vi "F510-X.vi"(8 "error in (no error)":errorcluster, 10 "Deadzone Scale Cluster":cluster{"Scale":dbl, "Deadzone":dbl}={"Scale"=1.0, "Deadzone"=0.1}, 11 "refnum name":string) -> (0 "error out":errorcluster, 1 "Right Stick":cluster{"X":dbl, "Y":dbl}, 2 "Left Stick":cluster{"X":dbl, "Y":dbl}, 3 "JoystickDevRef":T2, 4 "Buttons":T1, 5 "Triggers":cluster{"Left":dbl, "Right":dbl}, 6 "D-Pad Buttons":T4)   [LabVIEW 2014]
uses:
  <vilib>/Rock Robotics/WPI/Joystick/WPI_JoystickDevRef.ctl
  <vilib>/Rock Robotics/WPI/Joystick/WPI_JoystickDeviceEnum.ctl
  <vilib>/Rock Robotics/WPI/Joystick/WPI_JoystickGetSetRefNum.vi
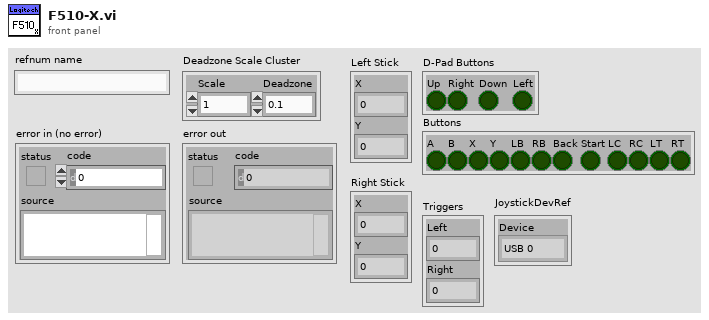
[diagram p1: front panel]
types:
  T1 = cluster{"A":bool, "B":bool, "X":bool, "Y":bool, "LB":bool, "RB":bool, "Back":bool, "Start":bool, "LC":bool, "RC":bool, "LT":bool, "RT":bool}
  T2 = typedef "WPI_JoystickDevRef.ctl" = cluster{"Device":T3}
  T3 = typedef "WPI_JoystickDeviceEnum.ctl" = enum16{"USB 0", "USB 1", "USB 2", "USB 3", "USB 4", "USB 5"}
  T4 = cluster{"Up":bool, "Right":bool, "Down":bool, "Left":bool}
  T5 = cluster{"[0]":dbl, "[1]":dbl, "[2]":dbl, "[3]":dbl, "[4]":dbl, "[5]":dbl}
  T6 = cluster{"Buttons[0]":bool, "Buttons[1]":bool, "Buttons[2]":bool, "Buttons[3]":bool, "Buttons[4]":bool, "Buttons[5]":bool, "Buttons[6]":bool, "Buttons[7]":bool, "Buttons[8]":bool, "Buttons[9]":bool}
  T7 = cluster{"Up":bool, "Down":bool, "Left":bool, "Right":bool}[]
  T8 = cluster{"Up":bool, "Down":bool, "Left":bool, "Right":bool}
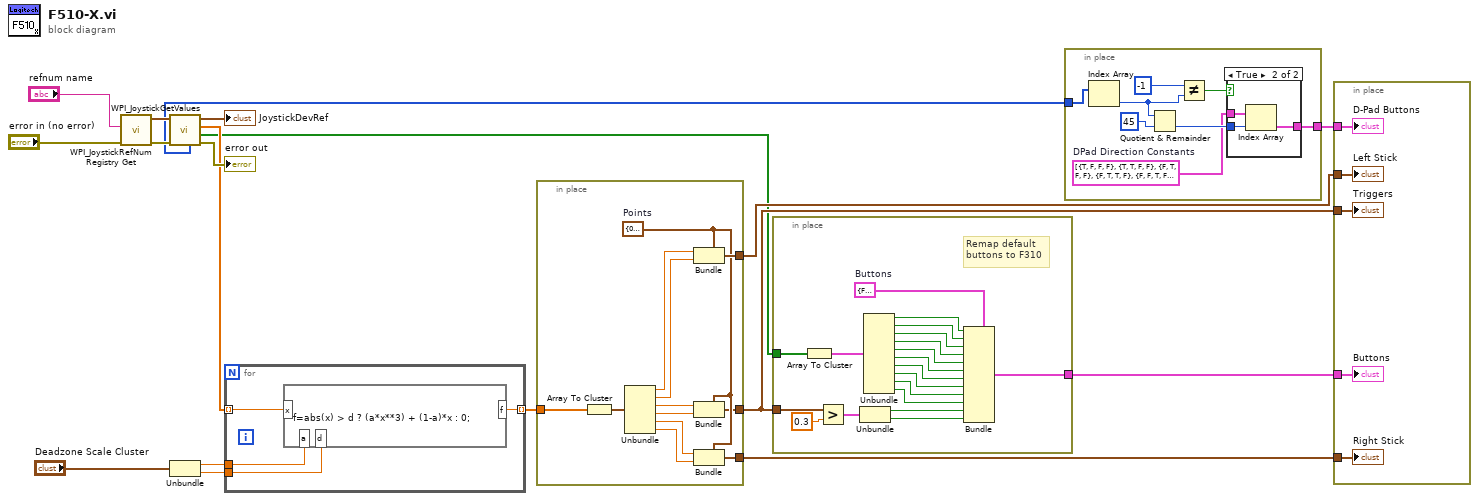
[diagram p0: block diagram]
diagram:
  n1 = call <vilib>:"WPI_JoystickRefNum Registry Get.vi"("error in (no error)"="error in (no error)", "refnum name"="refnum name") -> ("error out"=w15:errorcluster, "JoystickDevRef"=w16:T2)  [unwired: 8 in]
  n2 = call <vilib>:"WPI_JoystickGetValues.vi"("error in (no error)"=w15, "JoystickDevRef"=w16) -> ("error out"=→"error out":errorcluster, "Buttons"=w2:bool[], "Axes"=w13:dbl[], "JoystickDevRef"=→"JoystickDevRef":T2, "POVs"=w6:i16[])  [unwired: 5 in]
  n3 = Unbundle("Deadzone Scale Cluster") -> ("Scale"=w11:dbl, "Deadzone"=w10:dbl)
  n4 = for {
    tunnel: w13 -> [w22] mode=indexing
    tunnel: w11 -> [w21]
    tunnel: w10 -> [w20]
    tunnel: [w19] -> w9 mode=indexing
    n5 = formula code="f=abs(x) > d ? (a*x**3) + (1-a)*x : 0;"("x"=w22, "d"=w20, "a"=w21) -> ("f"=w19:dbl)
  }
  n6 = in-place {
    in-place-border: w9 -> [w31]
    in-place-border: [w27] -> w7
    in-place-border: [w30] -> w8
    in-place-border: [w25] -> w5
    w26 = cluster{"X":dbl, "Y":dbl} {"X"=0.0, "Y"=0.0}  # Points
    n7 = Array To Cluster(array=w31) -> (cluster=w34:T5)
    n8 = Unbundle(w34) -> ("[0]"=w32:dbl, "[1]"=w33:dbl, "[2]"=w24:dbl, "[3]"=w23:dbl, "[4]"=w29:dbl, "[5]"=w28:dbl)
    n9 = Bundle(cluster=w26, "X"=w32, "Y"=w33) -> (w30:cluster{"X":dbl, "Y":dbl})
    n10 = Bundle(cluster=w26, "X"=w24, "Y"=w23) -> (w25:cluster{"X":dbl, "Y":dbl})
    n11 = Bundle(cluster=w26, "X"=w29, "Y"=w28) -> (w27:cluster{"X":dbl, "Y":dbl})
  }
  n12 = in-place {
    in-place-border: w2 -> [w44]
    in-place-border: [w46] -> w1
    in-place-border: w5 -> [w39]
    w53 = T1 {"A"=FALSE, "B"=FALSE, "X"=FALSE, "Y"=FALSE, "LB"=FALSE, "RB"=FALSE, "Back"=FALSE, "Start"=FALSE, "LC"=FALSE, "RC"=FALSE, "LT"=FALSE, "RT"=FALSE}  # Buttons
    # "Remap default\nbuttons to F310"
    n13 = Array To Cluster(array=w44) -> (cluster=w45:T6)
    n14 = Greater?(x=w39, y=0.3) -> (0:w37:cluster{"X":bool, "Y":bool})
    n15 = Unbundle(w37) -> ("X"=w36:bool, "Y"=w35:bool)
    n16 = Unbundle(w45) -> ("Buttons[0]"=w52:bool, "Buttons[1]"=w51:bool, "Buttons[2]"=w50:bool, "Buttons[3]"=w49:bool, "Buttons[4]"=w48:bool, "Buttons[5]"=w47:bool, "Buttons[6]"=w43:bool, "Buttons[7]"=w42:bool, "Buttons[8]"=w41:bool, "Buttons[9]"=w40:bool)
    n17 = Bundle(cluster=w53, "A"=w52, "B"=w51, "X"=w50, "Y"=w49, "LB"=w48, "RB"=w47, "Back"=w43, "Start"=w42, "LC"=w41, "RC"=w40, "LT"=w36, "RT"=w35) -> (w46:T1)
  }
  n18 = in-place {
    in-place-border: w6 -> [w61]
    in-place-border: [w56] -> w4
    w57 = T7 [{"Up"=TRUE, "Down"=FALSE, "Left"=FALSE, "Right"=FALSE}, {"Up"=TRUE, "Down"=TRUE, "Left"=FALSE, "Right"=FALSE}, {"Up"=FALSE, "Down"=TRUE, "Left"=FALSE, "Right"=FALSE}, {"Up"=FALSE, "Down"=TRUE, "Left"=TRUE, "Right"=FALSE}, {"Up"=FALSE, "Down"=FALSE, "Left"=TRUE, "Right"=FALSE}, {"Up"=FALSE, "Down"=FALSE, "Left"=TRUE, "Right"=TRUE}, {"Up"=FALSE, "Down"=FALSE, "Left"=FALSE, "Right"=TRUE}, {"Up"=TRUE, "Down"=FALSE, "Left"=FALSE, "Right"=TRUE}]  # DPad Direction Constants
    n19 = Index Array(array=w61) -> (element=w55:i16)  [unwired: 1 in]
    n20 = Quotient & Remainder(x=w55, y=u16 45) -> (floor(x/y)=w59:u16)  [unwired: 1 out]
    n21 = Not Equal?(x=i16 -1, y=w55) -> (x != y?=w58:bool)
    n22 = case shown="True" w58 {
      tunnel: w59 -> [_ w64]
      tunnel: w57 -> [_ w63]
      tunnel: [_ w62] -> w56
      frame False {
      }
      frame True {
        n23 = Index Array(array=w63, index=w64) -> (element=w62:T8)
      }
    }
  }
  n24 = in-place {
    in-place-border: w8 -> [w69]
    in-place-border: w7 -> [w68]
    in-place-border: w5 -> [w67]
    in-place-border: w4 -> [w66]
    in-place-border: w1 -> [w65]
    "Left Stick" <- w69
    "Right Stick" <- w68
    "Triggers" <- w67
    "D-Pad Buttons" <- w66
    "Buttons" <- w65
  }
